vi "scan2d_destroy_UI_events.vi"(8 "error in (no error)":errorcluster, 11 "scan_panel in":refnum<class "scan_2d.lvclass">) -> (0 "error out":errorcluster, 3 "scan_panel out":refnum<class "scan_2d.lvclass">)   [LabVIEW 2015, in "scan_2d.lvclass"]
uses:
  scan_2d.lvclass
  scan_2d.lvclass/scan_2d.ctl
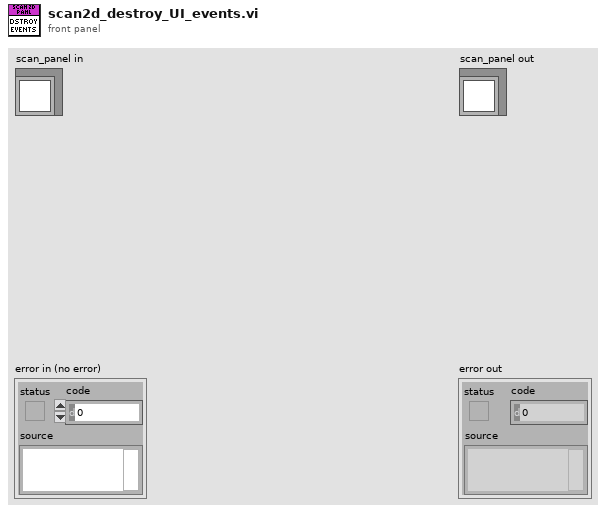
[diagram p1: front panel]
types:
  T1 = typedef "scan_ui_events.ctl" = cluster{"update_scan_status":refnum<user-event>}
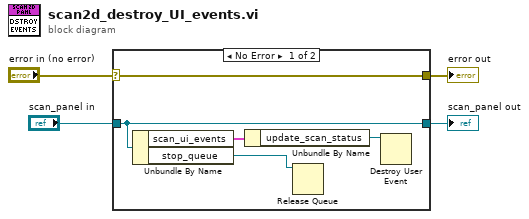
[diagram p0: block diagram]
diagram:
  n1 = case shown="No Error" "error in (no error)" {
    selector: "error in (no error)" -> [w9 w11]
    tunnel: [w9 w11] -> w3
    tunnel: [w8 w10] -> w1
    tunnel: "scan_panel in" -> [w8 w10]
    frame No Error {
      n2 = Unbundle By Name(w8) -> ("scan_ui_events"=w7:T1, "stop_queue"=w5:refnum<queue>)
      n3 = Unbundle By Name(w7) -> ("update_scan_status"=w6:refnum<user-event>)
      n4 = Release Queue(queue=w5) -> ()  [unwired: 2 in, 3 out]
      n5 = Destroy User Event(user event=w6) -> ()  [unwired: 1 in, 1 out]
    }
    frame Error {
    }
  }
  "error out" <- w3
  "scan_panel out" <- w1
